vi "CustomDriverStationTest.vi"   [LabVIEW 2017]
uses:
  <vilib>/Rock Robotics/Network Tables/NT Write Number.vi
  <vilib>/Rock Robotics/Network Tables/NT Write String.vi
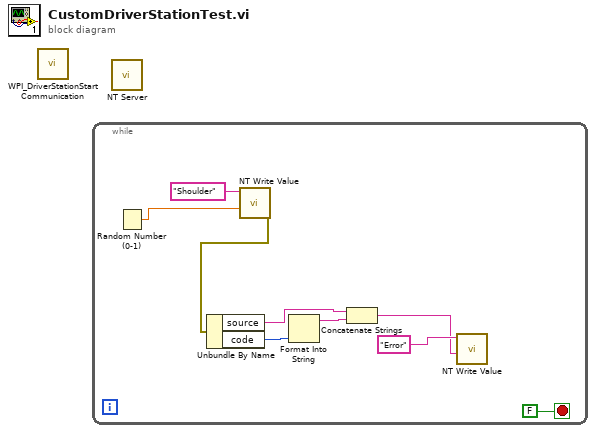
[diagram p0: block diagram]
diagram:
  n1 = call <vilib>:"WPI_DriverStationStart Communication.vi"() -> ()  [unwired: 2 in, 10 out]
  n2 = while {
    stop <- FALSE stop-if-true
    n3 = Random Number (0-1)() -> (number: 0 to 1=w8:dbl)
    n4 = call-poly <vilib>:"NT Write Value.vi"("Numeric"=w8, "Name"="Shoulder") -> ("error out"=w2:errorcluster)  [unwired: 9 in]
    n5 = Unbundle By Name(w2) -> ("source"=w3:string, "code"=w5:i32)
    n6 = Format Into String(w5) -> (resulting string=w4:string)  [unwired: 3 in, 1 out]
    n7 = Concatenate Strings(w3, w4) -> (w1:string)
    n8 = call-poly <vilib>:"NT Write Value.vi"("String"=w1, "Name"="Error") -> ()  [unwired: 9 in, 1 out]
  }
  n9 = call <vilib>:"NT Server.vi"() -> ()  [unwired: 12 in]
